vi "Read.vi"(8 "error out":errorcluster caption="error in", 10 "Read":T1={"Index"="``", "Sub-Index"="\u0000", "Data-Size (in Byte)"=1, FALSE} {"Data-Size (in Byte)" min=1 max=4 step=1 format="%x"}, 11 "ComPort In":refnum<visa-resource-name>="COM15") -> (0 "error out 2":errorcluster caption="error out", 2 "Answer":i32, 3 "ComPort Out":refnum<visa-resource-name>)   [LabVIEW 2021]
panel:
  out "read buffer":string
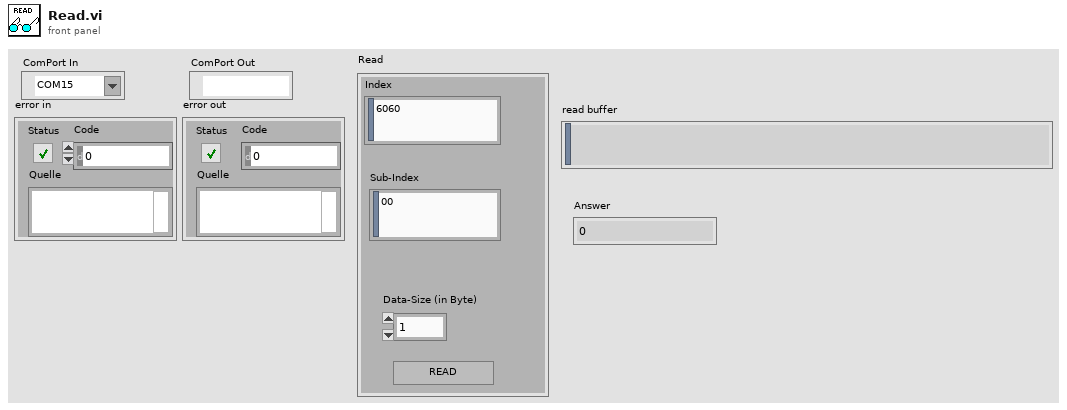
[diagram p1: front panel]
types:
  T1 = cluster{"Index":string, "Sub-Index":string, "Data-Size (in Byte)":u8, bool}
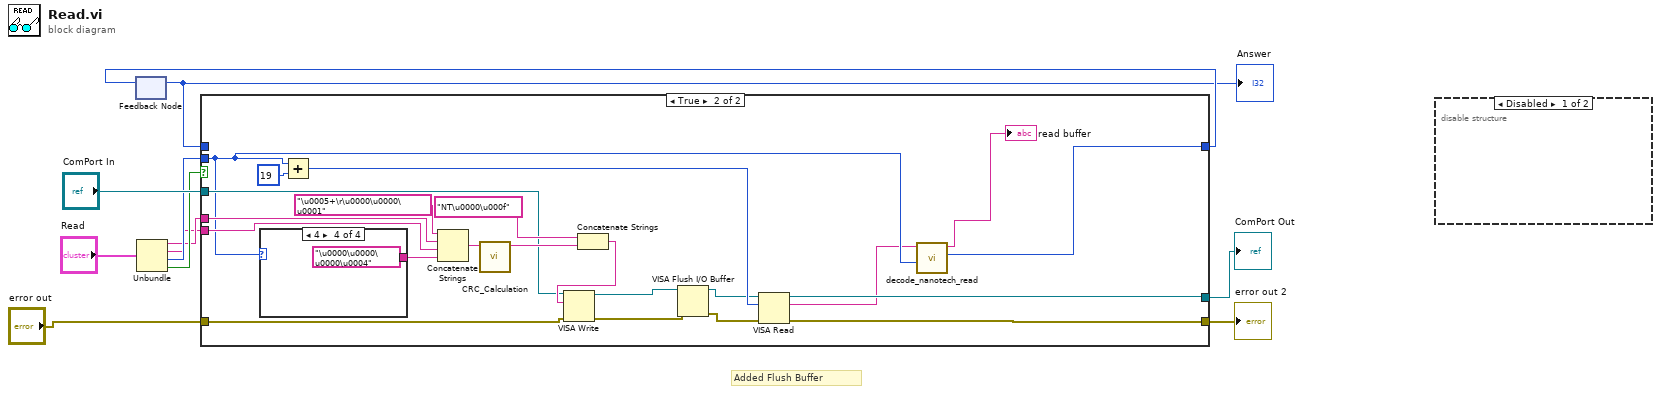
[diagram p0: block diagram]
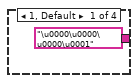
[diagram p4: hidden frame]
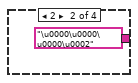
[diagram p5: hidden frame]
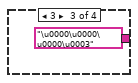
[diagram p6: hidden frame]
diagram:
  # "Added Flush Buffer"
  n1 = feedback #1() -> (w9:i32)  [unwired: 1 in]
  "Answer" <- w9
  n2 = Unbundle("Read") -> ("Index"=w3:string, "Sub-Index"=w2:string, "Data-Size (in Byte)"=w4:u8, w5:bool)
  n3 = case shown="True" w5 {
    tunnel: "ComPort In" -> [w13 w23]
    tunnel: "error out" -> [w14 w22]
    tunnel: [w14 w33] -> w11
    tunnel: w4 -> [_ w20]
    tunnel: w3 -> [_ w32]
    tunnel: w2 -> [_ w31]
    tunnel: [w13 w27] -> w7
    tunnel: [w12 w25] -> w10
    tunnel: w9 -> [w12 _]
    frame False {
    }
    frame True {
      n4 = case shown="4" w20 {
        tunnel: ["\u0000\u0000\u0000\u0001" ("Hexadecimal Input String 4") "\u0000\u0000\u0000\u0002" ("Hexadecimal Input String 4") "\u0000\u0000\u0000\u0003" ("Hexadecimal Input String 4") "\u0000\u0000\u0000\u0004" ("Hexadecimal Input String 4")] -> w26
        frame 1, Default {
        }
        frame 2 {
        }
        frame 3 {
        }
        frame 4 {
        }
      }
      n5 = Add(x=w20, y=u32 19 ("byte count")) -> (x+y=w28:u32)
      n6 = Concatenate Strings("\u0005+\r\u0000\u0000\u0001" ("Hexadecimal Input String 4"), w32, w31, w26) -> (w35:string)
      n7 = call "CRC_Calculation.vi"("CMD"=w35) -> ("CMD + CRC"=w34:string)  [unwired: 10 in]
      n8 = Concatenate Strings("NT\u0000\u000f" ("Hexadecimal Input String 4"), w34) -> (w24:string)
      n9 = VISA Write(VISA resource name=w23, write buffer=w24, error in (no error)=w22) -> (VISA resource name out=w18:refnum<visa-resource-name>, error out=w17:errorcluster)  [unwired: 1 out]
      n10 = VISA Flush I/O Buffer(VISA resource name=w18, error in (no error)=w17) -> (VISA resource name out=w16:refnum<visa-resource-name>, error out=w15:errorcluster)  [unwired: 1 in]
      n11 = VISA Read(VISA resource name=w16, byte count=w28, error in (no error)=w15) -> (VISA resource name out=w27:refnum<visa-resource-name>, read buffer=w19:string, error out=w33:errorcluster)  [unwired: 1 out]
      n12 = call "decode_nanotech_read.vi"("Data-Size (in Byte)"=w20, "read buffer in"=w19) -> ("Numeric Output"=w25:i32, "read buffer out"=→"read buffer":string)  [unwired: 8 in]
    }
  }
  "error out 2" <- w11
  "ComPort Out" <- w7
  n13 = feedback-in #1(w10) -> ()
  n14 = disable-structure shown="Disabled" {
    frame Disabled {
    }
    frame Enabled {
    }
  }
